vi "Configure Offset and Limits (Spectrum Emission Mask - RBW).vi"(0 "VISA resource name":refnum<visa-resource-name>, 1 "Manual Sweep Time List":dbl[](array[numeric])=[0.0075, 0.0075, 0.0075, 0.0075, 0.0075] format="%#.6g", 2 "Measurement Bandwidth List":i32[](array[numeric])=[1, 1, 1000, 1000, 1000], 5 "Auto Resolution Bandwidth List":bool[](array[boolean])=[FALSE, FALSE, FALSE, FALSE, FALSE], 7 "Manual Resolution Bandwidth List":dbl[](array[numeric])=[30000.0, 30000.0, 30000.0, 30000.0, 30000.0] format="%#.6g", 9 "Auto Sweep Time List":bool[](array[boolean])=[TRUE, TRUE, TRUE, TRUE, TRUE], 11 "error in (no error)":errorcluster) -> (4 "VISA resource name out":refnum<visa-resource-name>, 15 "error out":errorcluster)   [LabVIEW 2022 SP3, in "Agilent N934X Series.lvlib"]
doc: "Configures the RBW settings under the offsets and limits for Spectrum Emission Mask measurement type.\n\nNote:\nThis VI is only applicable for N9321C, N9322C, N9323C, N9324C models."
uses:
  <instrlib>/Agilent N934X Series/Agilent N934X Series.lvlib
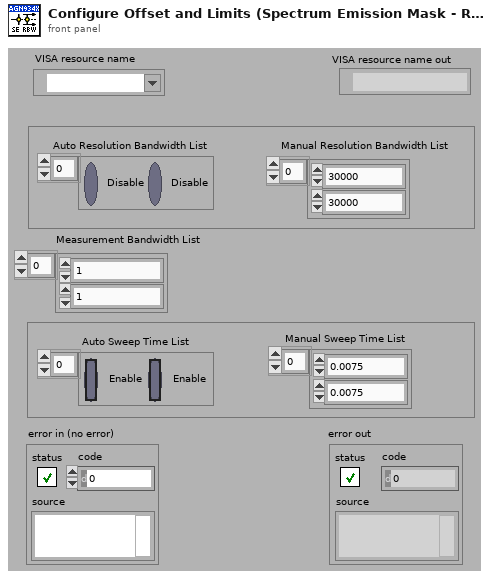
[diagram p1: front panel]
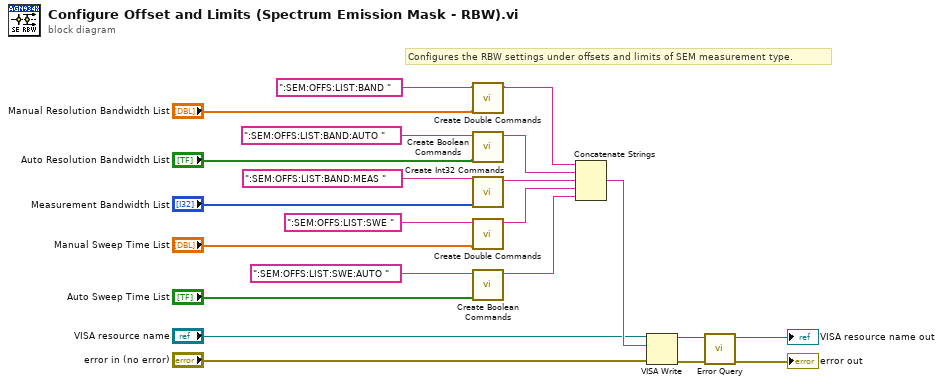
[diagram p0: block diagram]
diagram:
  # "Configures the RBW settings under offsets and limits of SEM measurement type."
  n1 = call <instrlib>:"Create Double Commands.vi"("Double Values"="Manual Resolution Bandwidth List", "Commands"=":SEM:OFFS:LIST:BAND " ("format string")) -> ("Result"=w5:string)  [unwired: 9 in]
  n2 = call <instrlib>:"Create Boolean Commands.vi"("Boolean States"="Auto Resolution Bandwidth List", "Command"=":SEM:OFFS:LIST:BAND:AUTO " ("format string")) -> ("Result String"=w10:string)  [unwired: 9 in]
  n3 = call <instrlib>:"Create Int32 Commands.vi"("Int Values"="Measurement Bandwidth List", "Commands"=":SEM:OFFS:LIST:BAND:MEAS " ("format string")) -> ("Result"=w17:string)  [unwired: 9 in]
  n4 = call <instrlib>:"Create Double Commands.vi"("Double Values"="Manual Sweep Time List", "Commands"=":SEM:OFFS:LIST:SWE " ("format string")) -> ("Result"=w9:string)  [unwired: 9 in]
  n5 = call <instrlib>:"Create Boolean Commands.vi"("Boolean States"="Auto Sweep Time List", "Command"=":SEM:OFFS:LIST:SWE:AUTO " ("format string")) -> ("Result String"=w8:string)  [unwired: 9 in]
  n6 = Concatenate Strings(w5, w10, w17, w9, w8) -> (w22:string)
  n7 = VISA Write(VISA resource name="VISA resource name", write buffer=w22, error in (no error)="error in (no error)") -> (VISA resource name out=w4:refnum<visa-resource-name>, error out=w3:errorcluster)  [unwired: 1 out]
  n8 = call <instrlib>:"Error Query.vi"("error in (no error)"=w3, "VISA resource name"=w4) -> ("error out"=→"error out":errorcluster, "VISA resource name out"=→"VISA resource name out":refnum<visa-resource-name>)  [unwired: 6 in, 2 out]
